vi "DisplayConfigDouble.vi"(9 "EnableSounds":bool) -> (4 "LovelaceIP":string, 6 "Cancelled?":bool, 8 "TeslaIP":string, 10 "EnableSounds out":bool, 15 "Score Behavior OUT":T1(ring))   [LabVIEW 2013]
uses:
  <vilib>/httpClient/LabVIEWHTTPClient.lvlib
panel:
  in  "Tab Control":enum32{"Page 1", "Page 2"}(tab)
  in  "Tab Control 2":enum32{"Basic Settings", "Advanced"}(tab)
  in  "Tesla":string="127.0.0.1"
  in  "Lovelace":string="127.0.0.1"
  in  "Check IP Button":bool
  in  "Port (ex:  8008)":string="8008"
  in  "Configure Sound Button":bool
  in  "Score Behavior":T1(ring)
  in  "Timer IP Addr":string="127.0.0.1"
  in  "MultiHomed Timer":bool
  in  "Process Stop Button":bool
  in  "OK Button":bool
  out "Instructions":string="This is the Display Application configuration utility for the FIRST LEGO League Tournament Software.  \n\nPlease type in the IP Address of the server system in the IP Address box to the left and press the \"Check\" button to verify that the server is running.  \"127.0.0.1\" is the default address for launching this application on the SERVER machine itself.  On the SERVER machine, the IP address can be found in the \"Monitor\" page at the bottom left.\n\nOnce you close this page, you can open this back up by pressing the ESC key.  You can press the SPACEBAR to make the display application expand the page, but the page MUST be on a display that is exactly 1024x768.\n\nThe display, by default, will show negative scores as ZERO while maintaining the negative value (for ranking purposes) within the software.  To show negatives scores at their true value, change the Score Behavior to reflect this.  \n\nThe display can play sounds similar to the server application.  This is a major hack, please only use this if you're using the standard sounds and don't need to change settings (unless you REALLY feel like you know what you're doing).  Currently sounds are only configured if enabled on initial launch of the display.  Sounds and config are NOT currently shared between the server and display, but the config information may be shared if hosted on the same computer.  Use with caution."
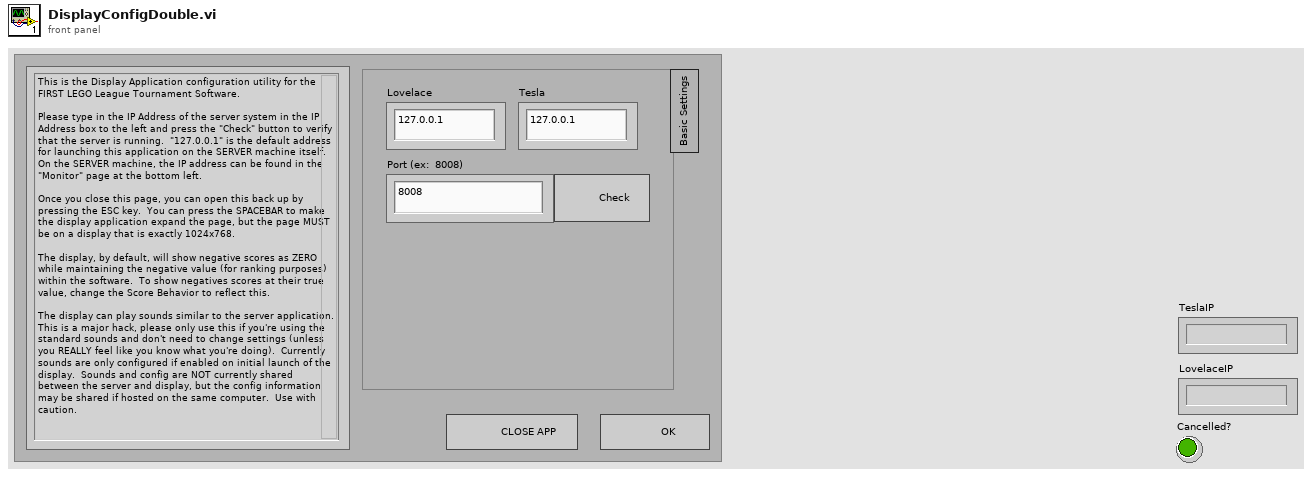
[diagram p1: front panel]
types:
  T1 = enum16{"Show Negative Scores as ZERO", "Show Negative Scores"}
  T2 = enum8{"Enabled", "Disabled", "Disabled and Grayed Out"}
  T3 = typedef "LabVIEWHTTPClient.lvlib/ClientHandle.ctl" = refnum<k1>
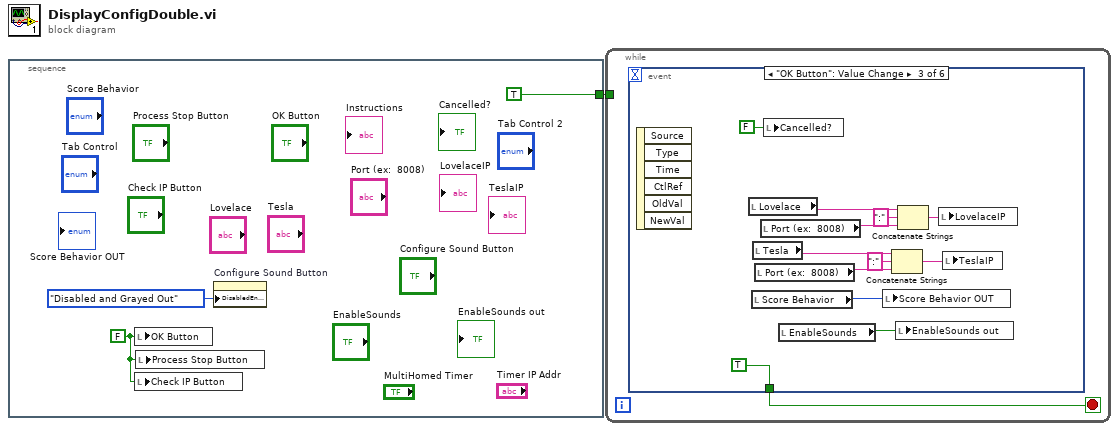
[diagram p0: block diagram]
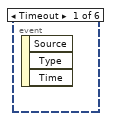
[diagram p2: hidden frame]
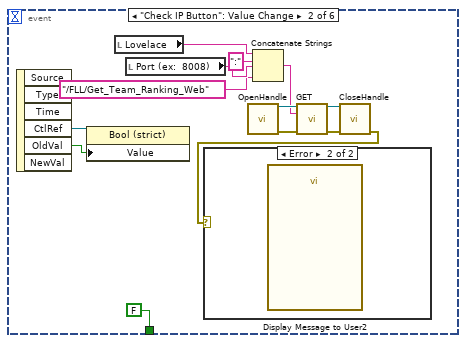
[diagram p3: hidden frame]
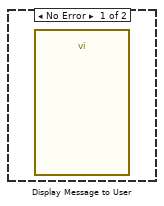
[diagram p4: hidden frame]
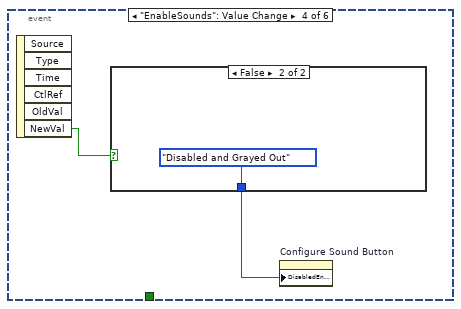
[diagram p5: hidden frame]
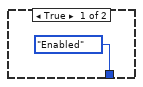
[diagram p6: hidden frame]
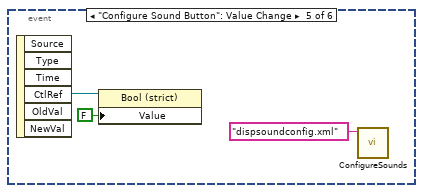
[diagram p7: hidden frame]
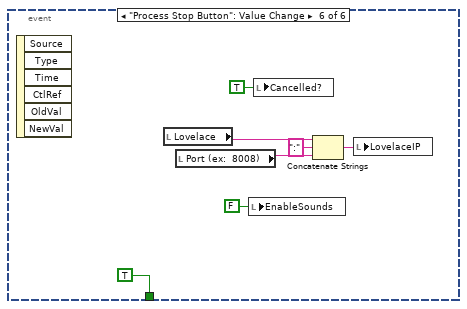
[diagram p8: hidden frame]
diagram:
  n1 = stacked-sequence {
    tunnel: [TRUE] -> w1
    frame #0 {
      w2 = FALSE ("OK Button")
      n2 = local write "OK Button"(w2) -> ()
      n3 = local write "Check IP Button"(w2) -> ()
      n4 = local write "Process Stop Button"(w2) -> ()
      n5 = property on="Configure Sound Button" class="Bool (strict)"("DisabledEnum"=T2."Disabled and Grayed Out" ("Disabled")) -> ()  [unwired: 2 in, 2 out]
    }
  }
  n6 = while {
    tunnel: w1 -> [_]
    stop <- w5 stop-if-true
    n7 = event shown="[2] \"OK Button\": Value Change" {
      selector: _ -> [_ _ _ _ _ _]
      dyn-events: _ -> [_ _ _ _ _ _]
      timeout: _ -> [_ _ _ _ _ _]
      tunnel: [_ FALSE TRUE _ _ TRUE] -> w5
      event Timeout {
        n8 = event-data() -> ()  [unwired: 1 in, 3 out]
      }
      event "Check IP Button": Value Change {
        n9 = event-data() -> ("CtlRef"=w16:refnum<vi>, "OldVal"=w15:bool)  [unwired: 1 in, 4 out]
        n10 = property class="Bool (strict)"(reference=w16, "Value"=w15) -> ()  [unwired: 1 in, 2 out]
        n11 = local read "Lovelace"() -> (w14:string)
        n12 = local read "Port (ex:  8008)"() -> (w12:string)
        n13 = call <vilib>:"OpenHandle.vi"() -> ("client handle out"=w18:T3, "error out"=w17:errorcluster)  [unwired: 14 in]
        n14 = Concatenate Strings(w14, ":" ("string"), w12, "/FLL/Get_Team_Ranking_Web" ("url")) -> (w10:string)
        n15 = call <vilib>:"GET.vi"("client handle"=w18, "url"=w10, "error in (no error)"=w17) -> ("client handle out"=w9:T3, "error out"=w8:errorcluster)  [unwired: 9 in, 2 out]
        n16 = call <vilib>:"CloseHandle.vi"("client handle"=w9, "error in (no error)"=w8) -> ("error out"=w7:errorcluster)  [unwired: 13 in]
        n17 = case shown="Error" w7 {
          frame No Error {
            n18 = call "Display Message to User"() -> ()  [unwired: 10 in, 2 out]
          }
          frame Error {
            n19 = call "Display Message to User2"() -> ()  [unwired: 10 in, 2 out]
          }
        }
      }
      event "OK Button": Value Change {
        n20 = event-data() -> ()  [unwired: 1 in, 6 out]
        n21 = local read "Lovelace"() -> (w29:string)
        n22 = local read "Score Behavior"() -> (w24:T1)
        n23 = local read "Tesla"() -> (w19:string)
        n24 = local read "Port (ex:  8008)"() -> (w20:string)
        n25 = local read "Port (ex:  8008)"() -> (w28:string)
        n26 = local write "Cancelled?"(FALSE ("Cancelled?")) -> ()
        n27 = local read "EnableSounds"() -> (w23:bool)
        n28 = local write "Score Behavior OUT"(w24) -> ()
        n29 = Concatenate Strings(w19, ":" ("string"), w20) -> (w22:string)
        n30 = local write "EnableSounds out"(w23) -> ()
        n31 = Concatenate Strings(w29, ":" ("string"), w28) -> (w26:string)
        n32 = local write "LovelaceIP"(w26) -> ()
        n33 = local write "TeslaIP"(w22) -> ()
      }
      event "EnableSounds": Value Change {
        n34 = event-data() -> ("NewVal"=w32:bool)  [unwired: 1 in, 5 out]
        n35 = case shown="False" w32 {
          tunnel: [T2."Enabled" ("Disabled") T2."Disabled and Grayed Out" ("Disabled")] -> w31
          frame True {
          }
          frame False {
          }
        }
        n36 = property on="Configure Sound Button" class="Bool (strict)"("DisabledEnum"=w31) -> ()  [unwired: 2 in, 2 out]
      }
      event "Configure Sound Button": Value Change {
        n37 = event-data() -> ("CtlRef"=w36:refnum<vi>)  [unwired: 1 in, 5 out]
        n38 = property class="Bool (strict)"(reference=w36, "Value"=FALSE) -> ()  [unwired: 1 in, 2 out]
        n39 = call "ConfigureSounds.vi"("File"="dispsoundconfig.xml") -> ()  [unwired: 9 in, 2 out]
      }
      event "Process Stop Button": Value Change {
        n40 = event-data() -> ()  [unwired: 1 in, 6 out]
        n41 = local read "Lovelace"() -> (w43:string)
        n42 = local read "Port (ex:  8008)"() -> (w42:string)
        n43 = local write "EnableSounds"(FALSE ("EnableSounds")) -> ()
        n44 = local write "Cancelled?"(TRUE ("Cancelled?")) -> ()
        n45 = Concatenate Strings(w43, ":" ("string"), w42) -> (w40:string)
        n46 = local write "LovelaceIP"(w40) -> ()
      }
    }
  }
